vi "0mqComm.vi"(10 "intercomm configuration":T1) -> (0 "last error":errorcluster)   [LabVIEW 2018]
uses:
  Custom/S4msg.ctl
  <vilib>/addons/zeromq/socket_type.ctl
  <vilib>/addons/zeromq/zeromq.lvlib
  <vilib>/addons/zeromq/zmq_context.lvclass
  <vilib>/addons/zeromq/zmq_socket.lvclass
panel:
  out "endpointPULL":string="localhost"
  out "last tick":u32
  out "endpointPUB":string="localhost"
  out "S4ICS_status":string caption="Status received from S4ICS"
  out "S4ICS_command":string caption="Command sent to S4ICS"
  in  "Stop Client":bool
  # "S4ICS 0mqCOMM"
  # "COMMUNICATION CHANNEL"
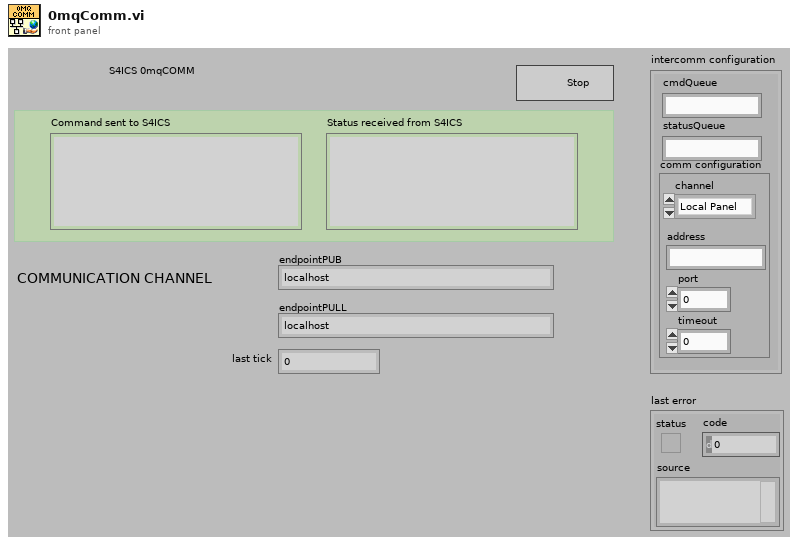
[diagram p1: front panel]
types:
  T1 = cluster{"S4commandQueueName":string, "S4statusQueueName":string, "comm configuration":cluster{"channel":enum32{"Local Panel", "Inner TCP/IP", "Outer TCP/IP", "MQTT", "ZeroMQ"}, "address":string, "port":u16, "timeout":i32}}
  T2 = typedef "zeromq.lvlib/socket_type.ctl" = enum8{"ZMQ_PAIR", "ZMQ_PUB", "ZMQ_SUB", "ZMQ_REQ", "ZMQ_REP", "ZMQ_DEALER", "ZMQ_ROUTER", "ZMQ_PULL", "ZMQ_PUSH", "ZMQ_XPUB", "ZMQ_XSUB", "ZMQ_STREAM", "ZMQ_SERVER", "ZMQ_CLIENT", "ZMQ_RADIO", "ZMQ_DISH", "ZMQ_GATHER", "ZMQ_SCATTER", "ZMQ_DGRAM"}
  T3 = typedef "S4msg.ctl" = cluster{"msg topic":string, "msg data":variant}
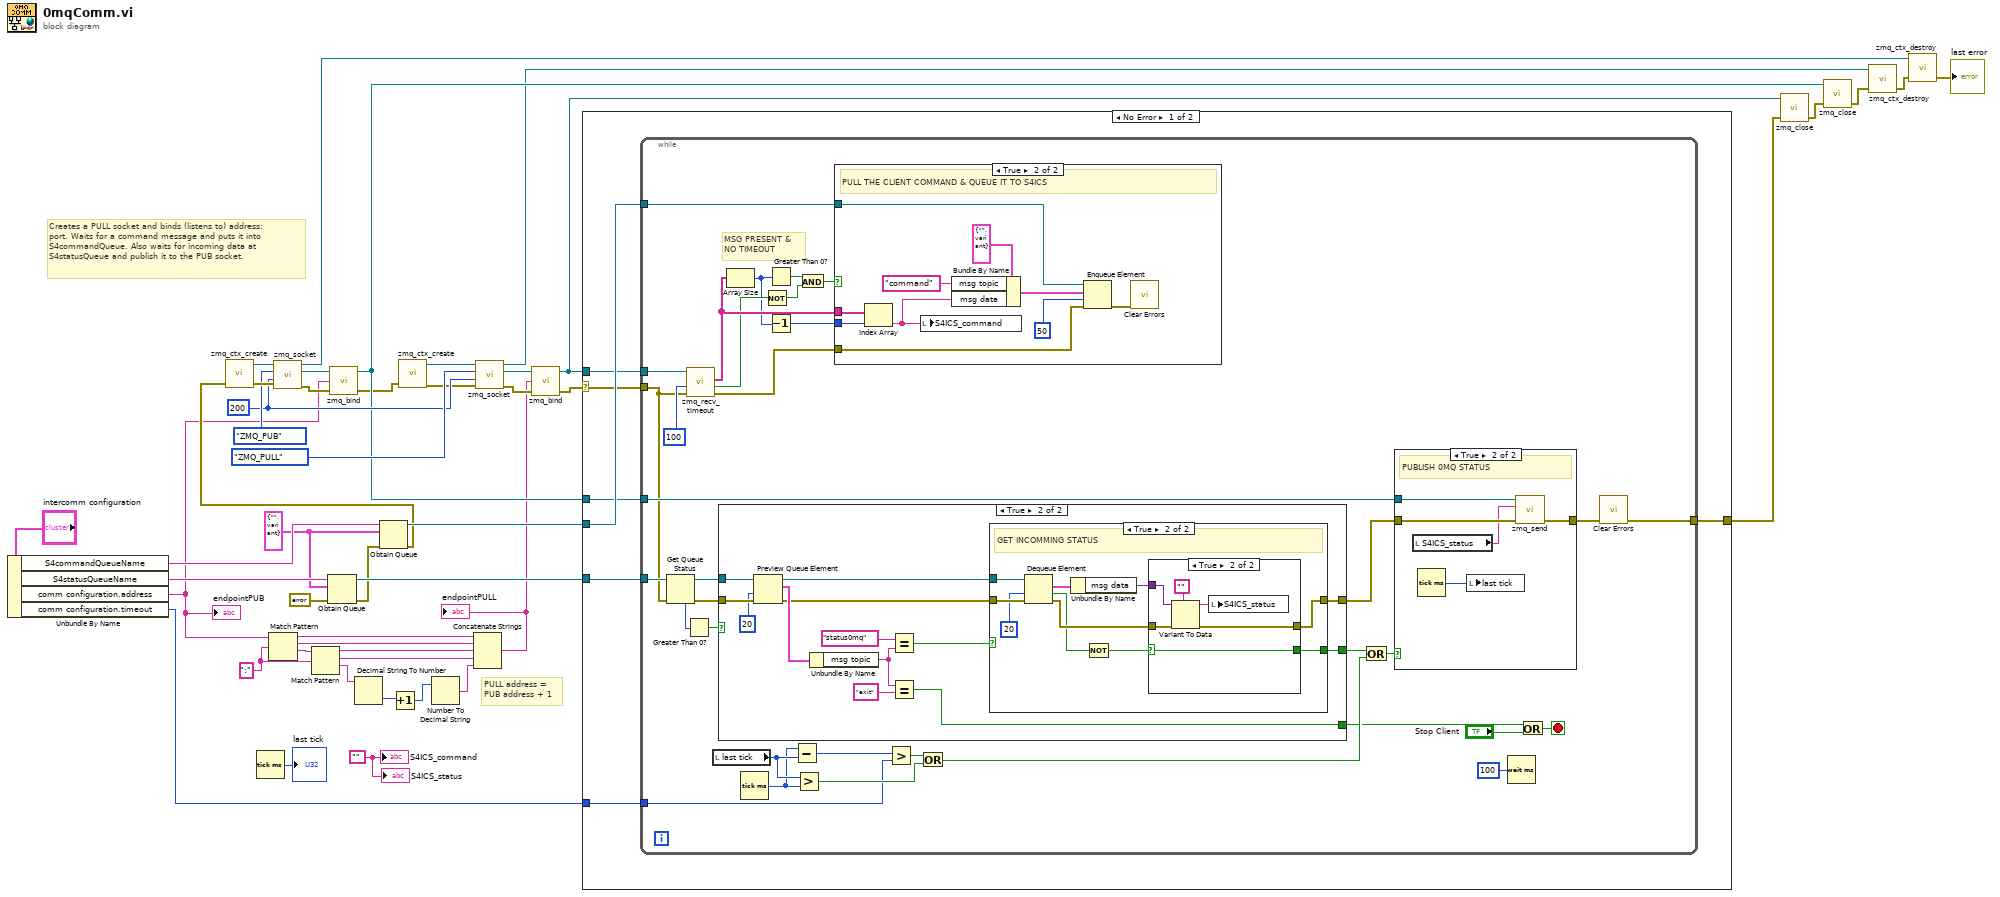
[diagram p0: block diagram]
diagram:
  w23 = 200 ("linger (ms)")
  w17 = ":" ("regular expression")
  w38 = T3 {"msg topic"="", "msg data"=variant} ("S4msg")
  w46 = ""
  # "PULL address =\nPUB address + 1"
  # "Creates a PULL socket and binds (listens to) address: port. Waits for a command message and puts it into S4commandQueue. Also waits for incoming data at S4statusQueue and publish it to the PUB socket."
  n1 = Unbundle By Name("intercomm configuration") -> ("S4commandQueueName"=w44:string, "S4statusQueueName"=w45:string, "comm configuration.address"=w2:string, "comm configuration.timeout"=w19:i32)
  "endpointPUB" <- w2
  n2 = Tick Count (ms)() -> (millisecond timer value=→"last tick":u32)
  n3 = Match Pattern(string=w2, regular expression=w17) -> (before substring=w25:string, match substring=w24:string, after substring=w18:string)  [unwired: 1 in, 1 out]
  n4 = Match Pattern(string=w18, regular expression=w17) -> (before substring=w15:string, match substring=w14:string, after substring=w13:string)  [unwired: 1 in, 1 out]
  n5 = Obtain Queue(name (unnamed)=w45, element data type=w38, error in (no error)=errorcluster {"status"=FALSE, "code"=0, "source"=""}) -> (queue out=w42:refnum<queue>, error out=w39:errorcluster)  [unwired: 2 in, 1 out]
  n6 = Decimal String To Number(string=w13) -> (number=w27:i32)  [unwired: 2 in, 1 out]
  n7 = Obtain Queue(name (unnamed)=w44, element data type=w38, error in (no error)=w39) -> (queue out=w43:refnum<queue>, error out=w41:errorcluster)  [unwired: 2 in, 1 out]
  n8 = call <vilib>:"zmq_ctx_create.vi"("error in"=w41) -> ("error out"=w36:errorcluster, "context out"=w30:refnum<class "zmq_context.lvclass">)  [unwired: 3 in]
  n9 = call <vilib>:"zmq_socket.vi"("error in"=w36, "linger (ms)"=w23, "socket type"=socket_type."ZMQ_PUB", "context in"=w30) -> ("error out"=w37:errorcluster, "socket out"=w34:refnum<class "zmq_socket.lvclass">, "context out"=w7:refnum<class "zmq_context.lvclass">)  [unwired: 1 in]
  n10 = call <vilib>:"zmq_bind.vi"("error in"=w37, "endpoint"=w2, "socket in"=w34) -> ("error out"=w4:errorcluster, "socket out"=w10:refnum<class "zmq_socket.lvclass">)  [unwired: 1 in]
  n11 = Increment(x=w27) -> (x+1=w26:i32)
  n12 = call <vilib>:"zmq_ctx_create.vi"("error in"=w4) -> ("error out"=w3:errorcluster, "context out"=w5:refnum<class "zmq_context.lvclass">)  [unwired: 3 in]
  n13 = Number To Decimal String(number=w26) -> (decimal integer string=w16:string)  [unwired: 1 in]
  n14 = Concatenate Strings(w25, w24, w15, w14, w16) -> (w1:string)
  "endpointPULL" <- w1
  n15 = call <vilib>:"zmq_socket.vi"("error in"=w3, "linger (ms)"=w23, "socket type"=socket_type."ZMQ_PULL", "context in"=w5) -> ("error out"=w33:errorcluster, "socket out"=w31:refnum<class "zmq_socket.lvclass">, "context out"=w8:refnum<class "zmq_context.lvclass">)  [unwired: 1 in]
  n16 = call <vilib>:"zmq_bind.vi"("error in"=w33, "endpoint"=w1, "socket in"=w31) -> ("error out"=w22:errorcluster, "socket out"=w20:refnum<class "zmq_socket.lvclass">)  [unwired: 1 in]
  n17 = case shown="No Error" w22 {
    selector: w22 -> [w49 w139]
    tunnel: w43 -> [w53 _]
    tunnel: w42 -> [w52 _]
    tunnel: w20 -> [w51 _]
    tunnel: w10 -> [w50 _]
    tunnel: [w48 w139] -> w21
    tunnel: w19 -> [w47 _]
    frame No Error {
      n18 = while {
        tunnel: [w63] -> w48
        tunnel: w53 -> [w68]
        tunnel: w52 -> [w87]
        tunnel: w51 -> [w75]
        tunnel: w50 -> [w79]
        tunnel: w49 -> [w64]
        tunnel: w47 -> [w59]
        stop <- w62 stop-if-true
        # "MSG PRESENT &\nNO TIMEOUT"
        n19 = Get Queue Status(queue=w87, error in (no error)=w64) -> (queue out=w58:refnum<queue>, error out=w57:errorcluster, # elements in queue=w55:i32)  [unwired: 1 in, 5 out]
        n20 = Greater Than 0?(x=w55) -> (x > 0?=w56:bool)
        n21 = call <vilib>:"zmq_recv_timeout.vi"("error in"=w64, "timeout (ms)"=u32 100, "socket in"=w75) -> ("error out"=w67:errorcluster, "timeout?"=w70:bool, "parts"=w73:string[])  [unwired: 1 in, 1 out]
        n22 = local read "last tick"() -> (w85:u32)
        n23 = case shown="True" w56 {
          selector: w56 -> [w88 _]
          tunnel: [w89 w102] -> w78
          tunnel: [w88 w101] -> w76
          tunnel: [w88 w90] -> w60
          tunnel: w58 -> [_ w100]
          tunnel: w57 -> [w89 w99]
          frame False {
          }
          frame True {
            n24 = Preview Queue Element(queue=w100, timeout in ms (-1)=20, error in (no error)=w99) -> (queue out=w95:refnum<queue>, element=w98:T3, error out=w94:errorcluster)  [unwired: 1 out]
            n25 = Unbundle By Name(w98) -> ("msg topic"=w91:string)
            n26 = Equal?(x="status0mq" ("msg topic"), y=w91) -> (x = y?=w96:bool)
            n27 = Equal?(x=w91, y="exit" ("msg topic")) -> (x = y?=w90:bool)
            n28 = case shown="True" w96 {
              selector: w96 -> [w103 _]
              tunnel: w94 -> [w104 w114]
              tunnel: w95 -> [_ w113]
              tunnel: [w104 w109] -> w102
              tunnel: [w103 w105] -> w101
              frame False {
              }
              frame True {
                # "GET INCOMMING STATUS"
                n29 = Dequeue Element(queue=w113, timeout in ms (-1)=20, error in (no error)=w114) -> (element=w112:T3, timed out?=w107:bool, error out=w110:errorcluster)  [unwired: 1 out]
                n30 = Unbundle By Name(w112) -> ("msg data"=w111:variant)
                n31 = Not(x=w107) -> (.not. x?=w106:bool)
                n32 = case shown="True" w106 {
                  selector: w106 -> [w116 w117]
                  tunnel: w111 -> [_ w122]
                  tunnel: w110 -> [w115 w121]
                  tunnel: [w115 w120] -> w109
                  tunnel: [w116 w117] -> w105
                  frame False {
                  }
                  frame True {
                    n33 = Variant To Data(error in=w121, type="", Variant=w122) -> (data=w118:string, error out=w120:errorcluster)
                    n34 = local write "S4ICS_status"(w118) -> ()
                  }
                }
              }
            }
          }
        }
        n35 = Array Size(array=w73) -> (size(s)=w66:i32)
        n36 = Tick Count (ms)() -> (millisecond timer value=w84:u32)
        n37 = Not(x=w70) -> (.not. x?=w71:bool)
        n38 = Greater Than 0?(x=w66) -> (x > 0?=w72:bool)
        n39 = Decrement(x=w66) -> (x-1=w65:i32)
        n40 = Subtract(x=w84, y=w85) -> (x-y=w86:u32)
        n41 = Greater?(x=w85, y=w84) -> (0:w82:bool)
        n42 = And(x=w72, y=w71) -> (x .and. y?=w69:bool)
        n43 = case shown="True" w69 {
          tunnel: w73 -> [_ w131]
          tunnel: w68 -> [_ w126]
          tunnel: w67 -> [_ w125]
          tunnel: w65 -> [_ w124]
          frame False {
          }
          frame True {
            # "PULL THE CLIENT COMMAND & QUEUE IT TO S4ICS"
            n44 = Index Array(array=w131, index=w124) -> (element=w128:string)
            n45 = local write "S4ICS_command"(w128) -> ()
            n46 = Bundle By Name(cluster=T3 {"msg topic"="", "msg data"=variant} ("S4msg"), "msg topic"="command", "msg data"=w128) -> (w127:T3)
            n47 = Enqueue Element(queue=w126, element=w127, timeout in ms (-1)=50, error in (no error)=w125) -> (error out=w123:errorcluster)  [unwired: 2 out]
            n48 = call <vilib>:"Clear Errors.vi"("error in (no error)"=w123) -> ()  [unwired: 5 in, 2 out]
          }
        }
        n49 = Greater?(x=w86, y=w59) -> (0:w83:bool)
        n50 = Or(x=w83, y=w82) -> (x .or. y?=w81:bool)
        n51 = Or(x=w76, y=w81) -> (x .or. y?=w80:bool)
        n52 = case shown="True" w80 {
          tunnel: [w133 w134] -> w77
          tunnel: w79 -> [_ w138]
          tunnel: w78 -> [w133 w137]
          frame False {
          }
          frame True {
            # "PUBLISH 0MQ STATUS"
            n53 = local read "S4ICS_status"() -> (w136:string)
            n54 = Tick Count (ms)() -> (millisecond timer value=w135:u32)
            n55 = local write "last tick"(w135) -> ()
            n56 = call <vilib>:"zmq_send.vi"("error in"=w137, "data"=w136, "socket in"=w138) -> ("error out"=w134:errorcluster)  [unwired: 4 in, 1 out]
          }
        }
        n57 = Wait (ms)(milliseconds to wait=u32 100) -> ()  [unwired: 1 out]
        n58 = Or(x=w60, y="Stop Client") -> (x .or. y?=w62:bool)
        n59 = call <vilib>:"Clear Errors.vi"("error in (no error)"=w77) -> ("error out"=w63:errorcluster)  [unwired: 5 in, 1 out]
      }
    }
    frame Error {
    }
  }
  n60 = call <vilib>:"zmq_close.vi"("error in"=w21, "socket"=w20) -> ("error out"=w12:errorcluster)  [unwired: 3 in]
  n61 = call <vilib>:"zmq_close.vi"("error in"=w12, "socket"=w10) -> ("error out"=w11:errorcluster)  [unwired: 3 in]
  n62 = call <vilib>:"zmq_ctx_destroy.vi"("error in"=w11, "context in"=w8) -> ("error out"=w9:errorcluster)  [unwired: 3 in]
  n63 = call <vilib>:"zmq_ctx_destroy.vi"("error in"=w9, "context in"=w7) -> ("error out"=→"last error":errorcluster)  [unwired: 3 in]
  "S4ICS_command" <- w46
  "S4ICS_status" <- w46
